vi "Ramp.vi"(0 "Enable":bool=TRUE, 1 "Start Value":dbl format="%#g", 2 "End Value":dbl format="%#g", 5 "error in (no error)":errorcluster) -> (16 "End Value":dbl format="%#g", 17 "Start Value":dbl format="%#g", 18 "OK":bool, 19 "error out":errorcluster)   [LabVIEW 2013]
doc: "Displays a standard dialog box that prompts users to enter information, such as a user name and password.\n--------------------\n\nThis Express VI is configured as follows:\n\nMessage to Display to the User:Enter start value and end value for ramp:\nThe inputs are: \nNumber: Start Value\nNumber: End Value"
panel:
  out "String":string="Enter start value and end value for ramp:"
  in  "Cancel":bool
  in  "OK2":bool
  in  "OK1":bool
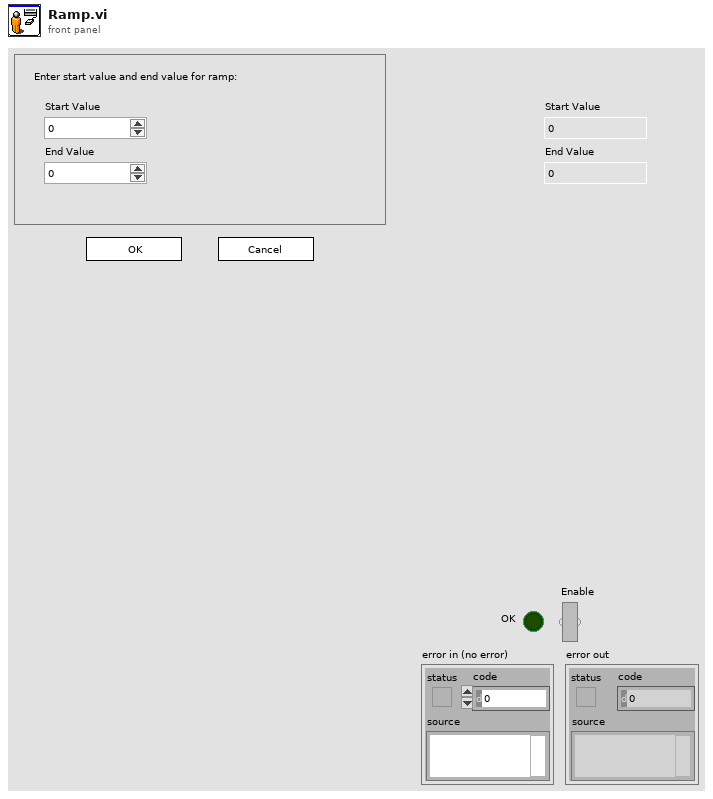
[diagram p1: front panel]
types:
  T1 = cluster{"Input Name":string, "Input Data Type":i32}[]
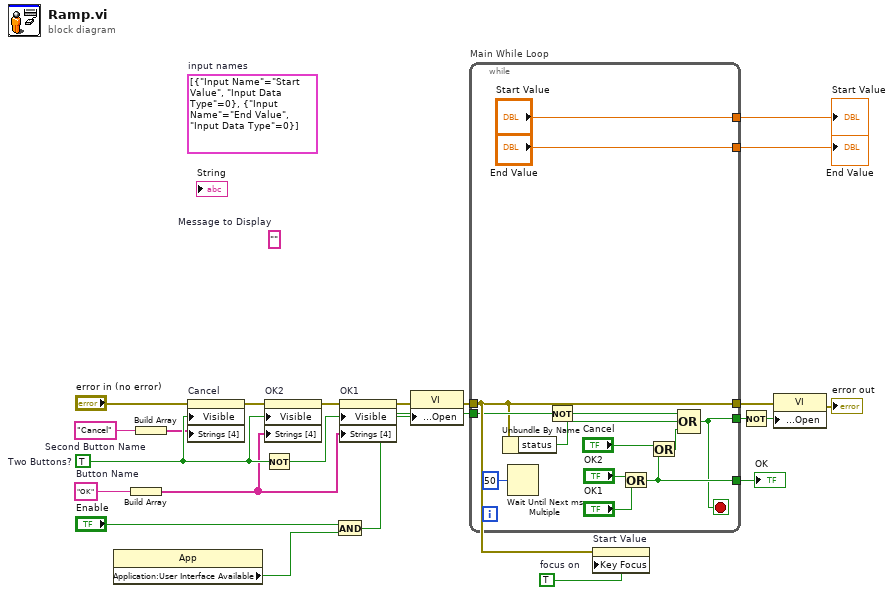
[diagram p0: block diagram]
diagram:
  w2 = TRUE  # focus on
  (unwired) T1 [{"Input Name"="Start Value", "Input Data Type"=0}, {"Input Name"="End Value", "Input Data Type"=0}]  # input names
  w14 = "Cancel"  # Second Button Name
  w12 = "OK"  # Button Name
  (unwired) ""  # Message to Display
  w22 = TRUE  # Two Buttons?
  n1 = property class="App"() -> ("Application:User Interface Available"=w4:bool)  [unwired: 2 in, 2 out]
  n2 = Build Array(w12) -> (w13:string[])
  n3 = Build Array(w14) -> (w15:string[])
  n4 = property on="Cancel" class="Bool"(error in="error in (no error)", "Visible"=w22, "Strings [4]"=w15) -> (error out=w19:errorcluster)  [unwired: 1 in, 1 out]
  n5 = Not(x=w22) -> (.not. x?=w20:bool)
  n6 = property on="OK2" class="Bool"(error in=w19, "Visible"=w22, "Strings [4]"=w13) -> (error out=w18:errorcluster)  [unwired: 1 in, 1 out]
  n7 = And(x="Enable", y=w4) -> (x .and. y?=w5:bool)
  n8 = property on="OK1" class="Bool"(error in=w18, "Visible"=w20, "Strings [4]"=w13) -> (error out=w11:errorcluster)  [unwired: 1 in, 1 out]
  n9 = property class="VI"(error in=w11, "Front Panel Window:Open"=w5) -> (error out=w10:errorcluster)  [unwired: 1 in, 1 out]
  n10 = while "Main While Loop" {
    tunnel: [w32] -> w21
    tunnel: w5 -> [w30]
    tunnel: [w28] -> w16
    tunnel: w10 -> [w27]
    tunnel: [w27] -> w8
    tunnel: ["Start Value"] -> w3
    tunnel: ["End Value"] -> w1
    stop <- w28 stop-if-true
    n11 = Unbundle By Name(w27) -> ("status"=w25:bool)
    n12 = Wait Until Next ms Multiple(millisecond multiple=u32 50) -> ()  [unwired: 1 out]
    n13 = Not(x=w30) -> (.not. x?=w29:bool)
    n14 = Or(x="OK2", y="OK1") -> (x .or. y?=w32:bool)
    n15 = Or(x="Cancel", y=w32) -> (x .or. y?=w26:bool)
    n16 = Compound Arithmetic op=OR(w29, w25, w26) -> (w28:bool)
  }
  "OK" <- w21
  "Start Value" <- w3
  "End Value" <- w1
  n17 = property on="Start Value" class="DigNum (strict)"(error in=w10, "Key Focus"=w2) -> ()  [unwired: 1 in, 2 out]
  n18 = Not(x=w16) -> (.not. x?=w17:bool)
  n19 = property class="VI"(error in=w8, "Front Panel Window:Open"=w17) -> (error out=→"error out":errorcluster)  [unwired: 1 in, 1 out]
